vi "EQ analysis.vi"(0 "number of pixels":u32, 5 "Condition over THLD sweep":bool, 7 "TOT (us)":u16=40, 9 "ADC target":u16=900, 11 "EQ Data and Report":u32[](array[numeric]) format="%x") -> (6 "EQ Data and Report, analyzed":u32[](array[numeric]) format="%x", 10 "quants pixels bons per Chip":u8[](array[numeric]))   [LabVIEW 2015, in "VIPM2.lvlib"]
doc: "<b>Equalization analysis</b>\nAnalitza els pixels d'una Layer (per Chip)\ni habilita (='0') els Triggers (PxReg[40]) dels pixels bons.\nEs programa només el cas d'una Layer."
uses:
  VIPM2.lvlib
panel:
  # "Equalization analysis"
  # "Analitza els pixels d'una Layer (per Chip)\ni habilita (='0') els Triggers (PxReg[40]) dels pixels bons"
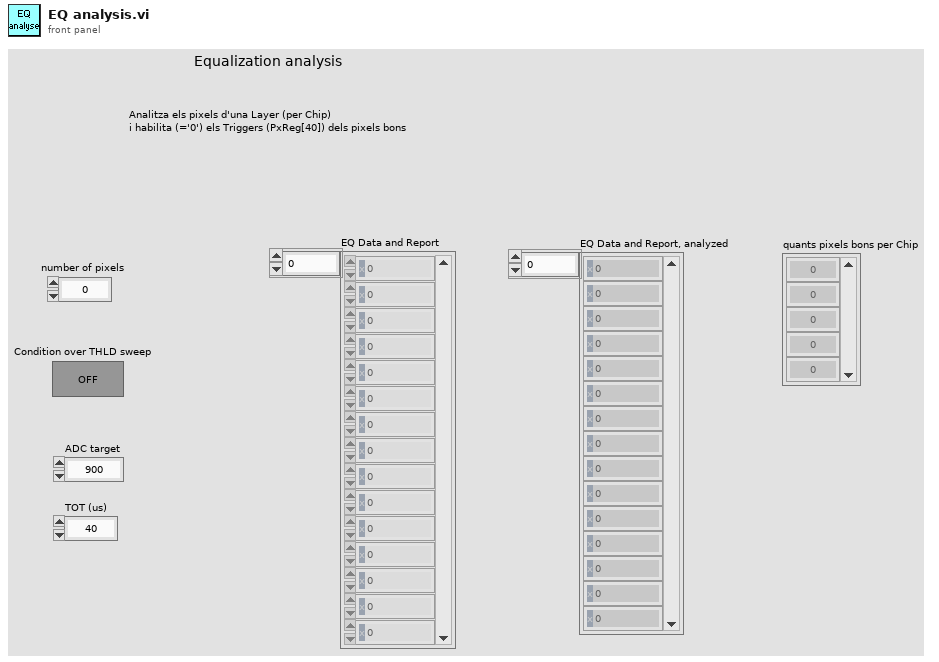
[diagram p1: front panel]
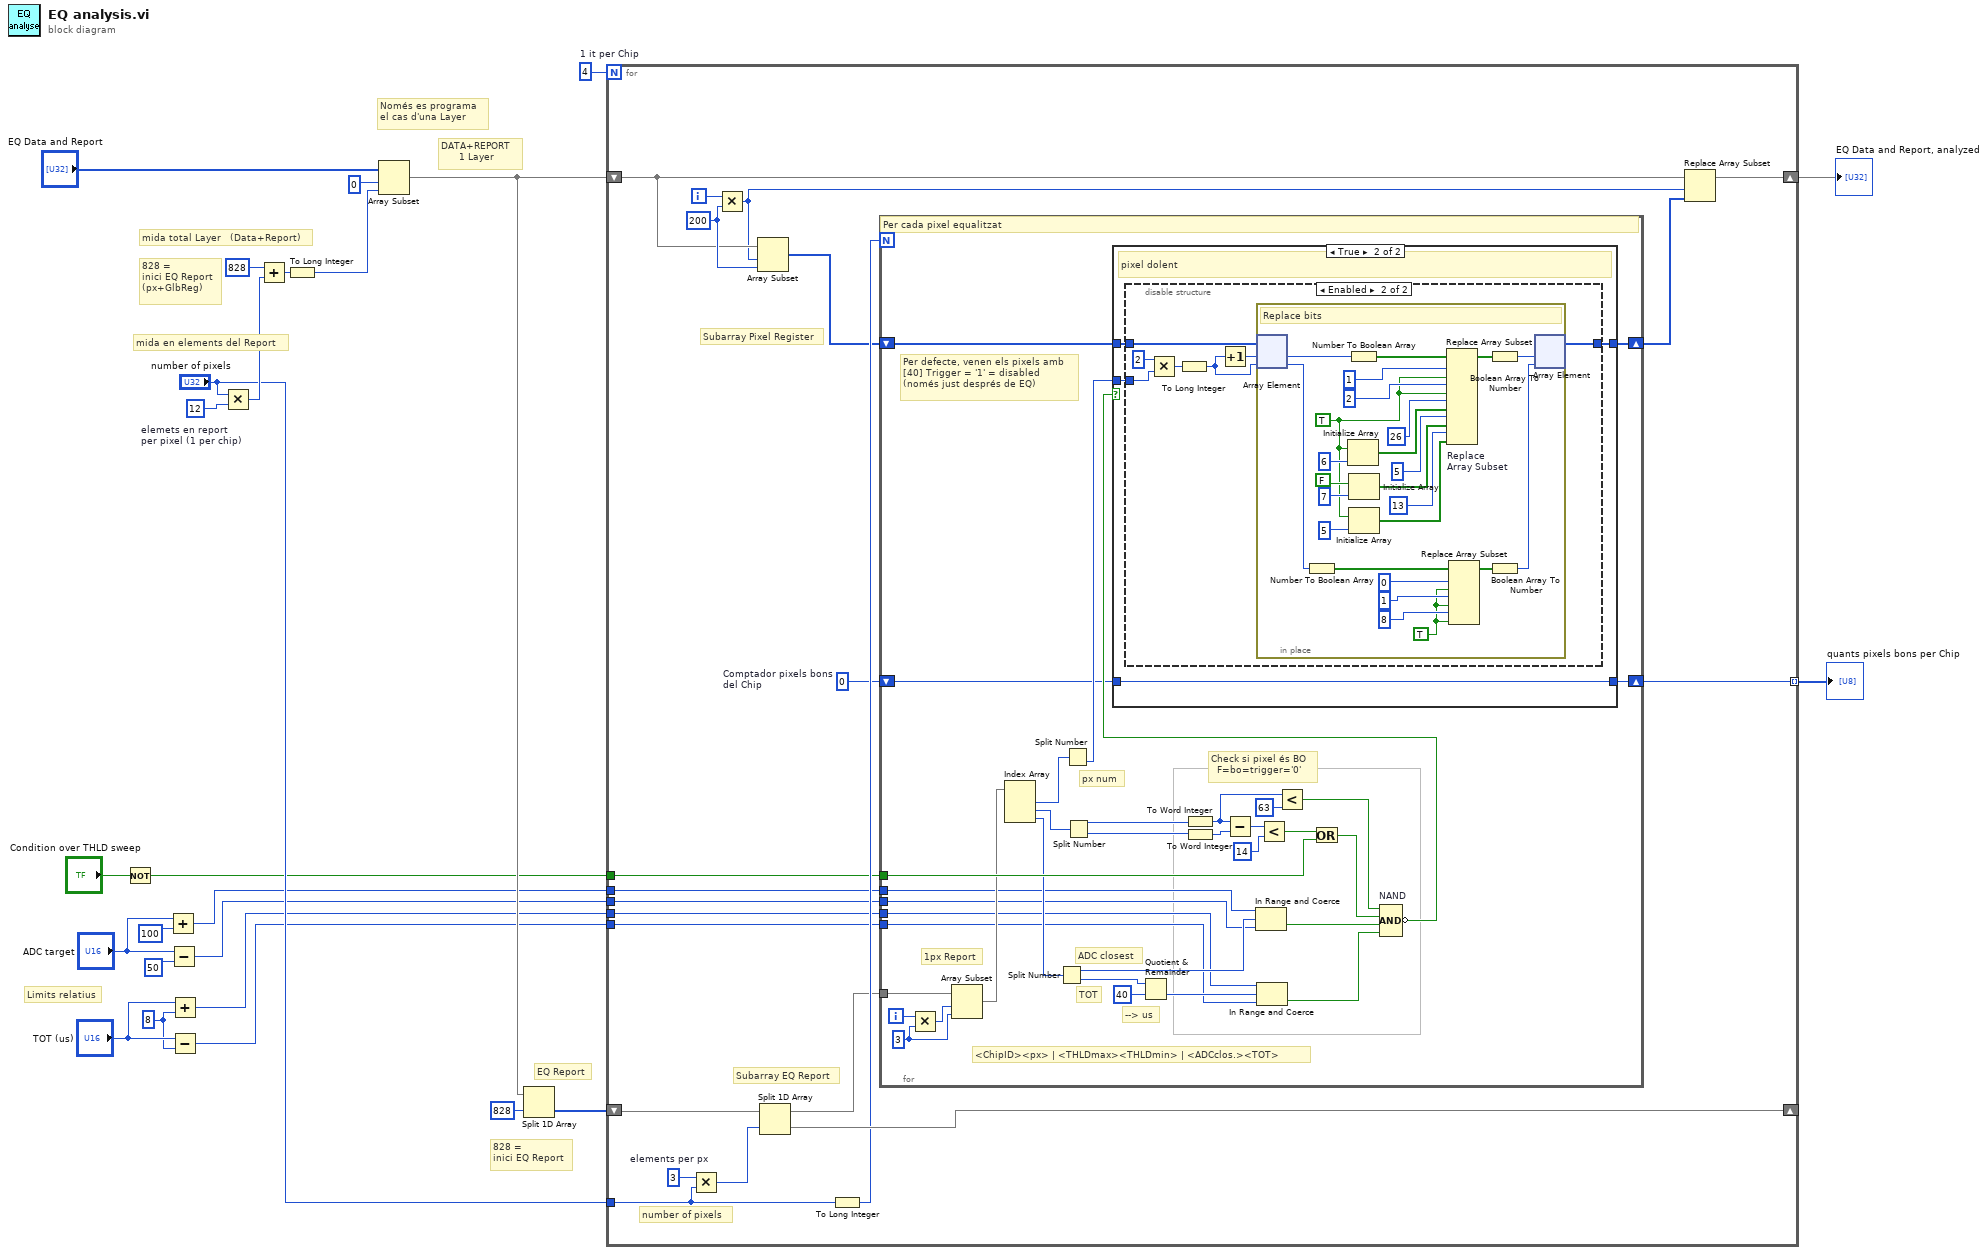
[diagram p0: block diagram]
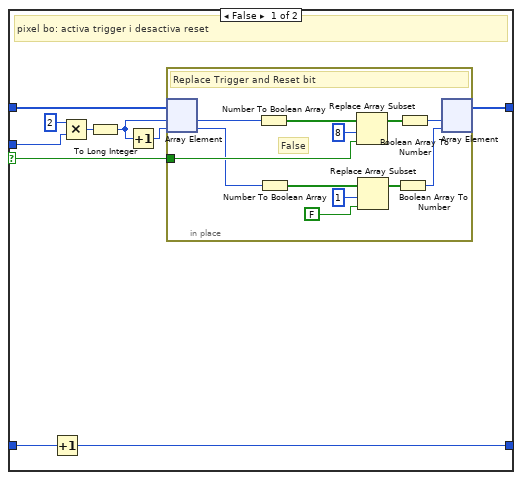
[diagram p2: hidden frame]
diagram:
  w3 = u16 8 ("y")
  w17 = 4  # 1 it per Chip
  w24 = u32 12  # elemets en report per pixel (1 per chip)
  # "Limits relatius"
  # "DATA+REPORT\n      1 Layer"
  # "EQ Report"
  # "828 =\ninici EQ Report"
  # "Només es programa\nel cas d'una Layer"
  # "mida total Layer   (Data+Report)"
  # "828 =\ninici EQ Report\n(px+GlbReg)"
  # "mida en elements del Report"
  n1 = Not(x="Condition over THLD sweep") -> (.not. x?=w10:bool)
  n2 = Add(x="ADC target", y=u16 100) -> (x+y=w6:u16)
  n3 = Subtract(x="ADC target", y=u16 50) -> (x-y=w5:u16)
  n4 = Add(x="TOT (us)", y=w3) -> (x+y=w2:u16)
  n5 = Subtract(x="TOT (us)", y=w3) -> (x-y=w1:u16)
  n6 = Multiply(x="number of pixels", y=w24) -> (x*y=w22:u32)
  n7 = Add(x=u32 828, y=w22) -> (x+y=w20:u32)
  n8 = To Long Integer(number=w20) -> (32bit integer=w19:i32)
  n9 = Array Subset "Array Subset"(array="EQ Data and Report", index=0, length=w19) -> (w14:u32[])
  n10 = Split 1D Array(array=w14, index=828) -> (second subarray=w16:u32[])  [unwired: 1 out]
  n11 = for {
    N: w17 -> [_]
    shift-right: [w45] -> _
    shift-left: w16 -> [w46]
    tunnel: "number of pixels" -> [w41]
    shift-right: [w34] -> w13
    shift-left: w14 -> [w36]
    tunnel: [w31] -> w12 mode=indexing
    tunnel: w10 -> [w30]
    tunnel: w6 -> [w29]
    tunnel: w5 -> [w28]
    tunnel: w2 -> [w27]
    tunnel: w1 -> [w26]
    i -> [w37]
    w32 = u8 0  # Comptador pixels bons del Chip
    w44 = u32 3  # elements per px
    w38 = 200 ("length")
    # "number of pixels"
    # "Subarray EQ Report"
    # "Subarray Pixel Register"
    n12 = Multiply(x=w44, y=w41) -> (x*y=w43:u32)
    n13 = Multiply(x=w37, y=w38) -> (x*y=w35:i32)
    n14 = Array Subset "Array Subset"(array=w36, index=w35, length=w38) -> (w39:u32[])
    n15 = Split 1D Array(array=w46, index=w43) -> (first subarray=w40:u32[], second subarray=w45:u32[])
    n16 = To Long Integer(number=w41) -> (32bit integer=w42:i32)
    n17 = for {
      N: w42 -> [_]
      tunnel: w40 -> [w79]
      shift-right: [w66] -> w33
      shift-left: w39 -> [w71]
      shift-right: [w59] -> w31
      shift-left: w32 -> [w60]
      tunnel: w30 -> [w81]
      tunnel: w29 -> [w50]
      tunnel: w28 -> [w49]
      tunnel: w27 -> [w48]
      tunnel: w26 -> [w47]
      i -> [w80]
      w77 = 3 ("y")
      # "--> us"
      # "Per defecte, venen els pixels amb\n[40] Trigger = '1' = disabled\n(només just després de EQ)"
      # "Check si pixel és BO\n  F=bo=trigger='0'"
      # "TOT"
      # "ADC closest"
      # "px num"
      # "<ChipID><px> | <THLDmax><THLDmin> | <ADCclos.><TOT>"
      # "1px Report"
      # "Per cada pixel equalitzat"
      n18 = Multiply(x=w80, y=w77) -> (x*y=w78:i32)
      n19 = Array Subset "Array Subset"(array=w79, index=w78, length=w77) -> (w76:u32[])
      n20 = Index Array "Index Array"(array=w76) -> (element #1=w75:u32, element #2=w74:u32, element #3=w73:u32)  [unwired: 3 in]
      n21 = Split Number(x=w73) -> (hi(x)=w72:u16, lo(x)=w65:u16)
      n22 = Split Number(x=w75) -> (lo(x)=w70:u16)  [unwired: 1 out]
      n23 = Split Number(x=w74) -> (hi(x)=w62:u16, lo(x)=w61:u16)
      n24 = Quotient & Remainder(x=w65, y=u16 40) -> (floor(x/y)=w63:u16)  [unwired: 1 out]
      n25 = To Word Integer(number=w62) -> (16bit integer=w53:i16)
      n26 = To Word Integer(number=w61) -> (16bit integer=w58:i16)
      n27 = Subtract(x=w53, y=w58) -> (x-y=w57:i16)
      n28 = In Range and Coerce(upper limit=w50, x=w72, lower limit=w49) -> (In Range?=w68:bool)  [unwired: 1 out]
      n29 = In Range and Coerce(upper limit=w48, x=w63, lower limit=w47) -> (In Range?=w67:bool)  [unwired: 1 out]
      n30 = Less?(x=w57, y=i16 14) -> (x < y?=w55:bool)
      n31 = Less?(x=w53, y=i16 63) -> (x < y?=w51:bool)
      n32 = Or(x=w55, y=w81) -> (x .or. y?=w54:bool)
      n33 = Compound Arithmetic op=AND "NAND"(w51, w54, w68, w67) -> (invert w69:bool)
      n34 = case shown="True" w69 {
        selector: w69 -> [w87 _]
        tunnel: w71 -> [w91 w105]
        tunnel: w70 -> [w88 w104]
        tunnel: [w86 w106] -> w66
        tunnel: w60 -> [w85 w107]
        tunnel: [w84 w107] -> w59
        frame False {
          # "pixel bo: activa trigger i desactiva reset"
          n35 = Increment(x=w85) -> (x+1=w84:u8)
          n36 = Multiply(x=u16 2, y=w88) -> (x*y=w89:u16)
          n37 = To Long Integer(number=w89) -> (32bit integer=w83:i32)
          n38 = Increment(x=w83) -> (x+1=w82:i32)
          n39 = in-place {
            in-place-border: w87 -> [w98]
            # "False"
            # "Replace Trigger and Reset bit"
            n40 = in-place-array #1(w91, w83, w82) -> (w103:u32, w95:u32)
            n41 = Number To Boolean Array(number=w103) -> (Boolean array=w102:bool[])
            n42 = Number To Boolean Array(number=w95) -> (Boolean array=w96:bool[])
            n43 = Replace Array Subset(array=w102, new element=w98, index=8) -> (w100:bool[])
            n44 = Replace Array Subset(array=w96, new element=FALSE, index=1) -> (w93:bool[])
            n45 = Boolean Array To Number(Boolean array=w93) -> (number=w92:u32)
            n46 = Boolean Array To Number(Boolean array=w100) -> (number=w99:u32)
            n47 = in-place-array #1(w99, w92) -> (w86:u32[])  [unwired: 2 out]
          }
        }
        frame True {
          # "pixel dolent"
          n48 = disable-structure shown="Enabled" {
            disable-tunnel: [w108 w112] -> w106
            disable-tunnel: w105 -> [w108 w113]
            disable-tunnel: w104 -> [_ w111]
            frame Disabled {
            }
            frame Enabled {
              n49 = Multiply(x=u16 2, y=w111) -> (x*y=w114:u16)
              n50 = To Long Integer(number=w114) -> (32bit integer=w109:i32)
              n51 = Increment(x=w109) -> (x+1=w110:i32)
              n52 = in-place {
                w120 = TRUE
                w118 = TRUE
                # "Replace bits"
                n53 = in-place-array #2(w113, w110, w109) -> (w140:u32, w127:u32)
                n54 = Number To Boolean Array(number=w127) -> (Boolean array=w126:bool[])
                n55 = Initialize Array(w118, 6 ("dimension size")) -> (w131:bool[])
                n56 = Number To Boolean Array(number=w140) -> (Boolean array=w139:bool[])
                n57 = Initialize Array(FALSE, 7 ("dimension size")) -> (w133:bool[])
                n58 = Initialize Array(w118, 5 ("dimension size")) -> (w116:bool[])
                n59 = Replace Array Subset "Replace \nArray Subset"(array=w139, new element #1=w118, index #1=1 ("index"), new element #2=w118, index #2=2 ("index"), new element #3=w131, index #3=26 ("index"), new element #4=w133, index #4=5 ("index"), new element #5=w116, index #5=13 ("index")) -> (w138:bool[])
                n60 = Replace Array Subset(array=w126, new element #1=w120, index #1=0 ("index"), new element #2=w120, index #2=1 ("index"), new element #3=w120, index #3=8 ("index")) -> (w125:bool[])
                n61 = Boolean Array To Number(Boolean array=w138) -> (number=w137:u32)
                n62 = Boolean Array To Number(Boolean array=w125) -> (number=w124:u32)
                n63 = in-place-array #2(w137, w124) -> (w112:u32[])  [unwired: 2 out]
              }
            }
          }
        }
      }
    }
    n64 = Replace Array Subset "Replace Array Subset"(array=w36, new element=w33, index=w35) -> (w34:u32[])
  }
  "EQ Data and Report, analyzed" <- w13
  "quants pixels bons per Chip" <- w12
